vi "ProcessingLoop.vi"(8 "error in (no error)":errorcluster, 11 "navX - Base in":refnum<class "navX - Base.lvclass">) -> (0 "error out":errorcluster, 3 "navX - Base out":refnum<class "navX - Base.lvclass">)   [LabVIEW 2015, in "navX Library v3.lvlib" / "navX - Base.lvclass"]
uses:
  navX - Base.lvclass
  navX Error Status/navX Error Status.lvclass
  navX - Base.lvclass/navX - Base.ctl
  <vilib>/Platform/TimedLoop/XDataNode/timing_clust.ctl
  <vilib>/Platform/TimedLoop/XDataNode/nitl_modes.ctl
  <vilib>/Platform/TimedLoop/XDataNode/wakeup.ctl
  <vilib>/platform/TimedLoop/XDataNode/XDataNode.xnode
  <vilib>/Platform/TimedLoop/XDataNode/XDNodeRunTimeDep.lvlib
panel:
  out "Iteration Duration":i64
  out "Finished Late? [i-1]":bool
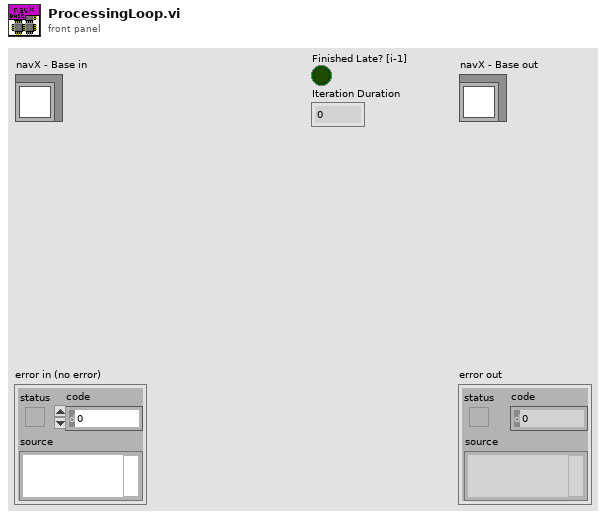
[diagram p1: front panel]
types:
  T1 = typedef "XDNodeRunTimeDep.lvlib/timing_clust.ctl" = cluster{"Expected End [f-1]":u64, "Actual End [f-1]":u64, "Finished Late? [f-1]":bool, "Expected End [i-1]":u64, "Actual End [i-1]":u64, "Finished Late? [i-1]":bool, "Expected Start [i]":u64, "Actual Start [i]":u64, "Expected Start [f]":u64, "Actual Start [f]":u64, "Source Name":string, "Structure Name":string, "Period":i64, "Deadline":i64, "Offset":i64, "Start":i64, "Priority":i32, "Timeout":i32, "Mode":T2, "Wakeup Reason":T3, "Error":errorcluster, "Source Type":string, "Secondary Source Type":string, "Global End Time":u64, "Global Start Time":u64, "Frame Duration":u64, "Iteration Duration":u64, "Assigned CPU":i32, "I/O Scan Engine Mode":u32}
  T2 = typedef "XDNodeRunTimeDep.lvlib/nitl_modes.ctl" = enum32{"No Change", "Process missed periods, maintain original phase", "Discard missed periods, maintain original phase", "Process missed periods, ignore original phase", "Discard missed periods, ignore original phase"}
  T3 = typedef "XDNodeRunTimeDep.lvlib/wakeup.ctl" = enum32{"Normal", "Aborted", "Asynchronous wakeup", "Timing source error", "Timed loop error", "Timeout"}
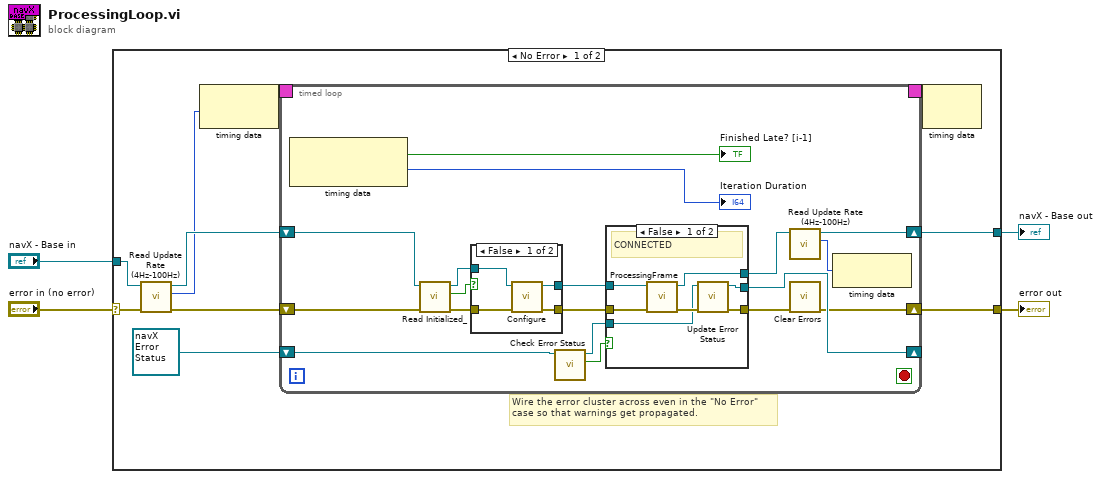
[diagram p0: block diagram]
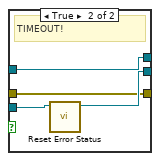
[diagram p3: hidden frame]
diagram:
  n1 = case shown="No Error" "error in (no error)" {
    selector: "error in (no error)" -> [w7 w61]
    tunnel: [w6 w61] -> w3
    tunnel: [w10 w60] -> w1
    tunnel: "navX - Base in" -> [w12 w60]
    frame No Error {
      # "Wire the error cluster across even in the \"No Error\"\ncase so that warnings get propagated."
      n2 = call "Read Update Rate (4Hz-100Hz).vi"("error in (no error)"=w7, "navX - Base in"=w12) -> ("error out"=w9:errorcluster, "Update Rate (4Hz-100Hz)"=w5:u8, "navX - Base out"=w11:refnum<class "navX - Base.lvclass">)  [unwired: 7 in]
      n3 = node-c288(w5) -> (w14:T1)
      n4 = timed-loop {
        timing: w14 -> [_]
        timing-out: [_] -> w13
        shift-right: [w32] -> w10
        shift-left: w11 -> [w21]
        shift-right: [w24] -> w6
        shift-left: w9 -> [w20]
        shift-right: [w27] -> _
        shift-left: refnum<class "navX Error Status.lvclass"> refnum ("navX Library v3.lvlib:navX Error Status.lvclass") -> [w30]
        stop <- _ stop-if-true
        n5 = node-c288() -> (→"Finished Late? [i-1]":bool, →"Iteration Duration":i64)  [unwired: 1 in]
        n6 = call "Read Initialized_.vi"("error in (no error)"=w20, "navX - Base in"=w21) -> ("error out"=w17:errorcluster, "Initialized?"=w18:bool, "navX - Base out"=w19:refnum<class "navX - Base.lvclass">)  [unwired: 7 in]
        n7 = case shown="False" w18 {
          tunnel: [w36 w37] -> w23
          tunnel: [w35 w38] -> w22
          tunnel: w19 -> [w34 w38]
          tunnel: w17 -> [w33 w37]
          frame False {
            n8 = call-dynamic "Configure.vi"("error in (no error)"=w33, "navX - Base in"=w34) -> ("error out"=w36:errorcluster, "navX - Base out"=w35:refnum<class "navX - Base.lvclass">)  [unwired: 8 in]
          }
          frame True {
          }
        }
        n9 = call "Check Error Status.vi"("navX Error Status in"=w30) -> ("Timeout!"=w29:bool, "navX Error Status out"=w28:refnum<class "navX Error Status.lvclass">)  [unwired: 8 in, 1 out]
        n10 = case shown="False" w29 {
          tunnel: w28 -> [w42 w49]
          tunnel: w22 -> [w45 w47]
          tunnel: w23 -> [w44 w46]
          tunnel: [w41 w48] -> w27
          tunnel: [w40 w46] -> w25
          tunnel: [w39 w47] -> w26
          frame False {
            # "CONNECTED"
            n11 = call-dynamic "ProcessingFrame.vi"("error in (no error)"=w44, "navX - Base in"=w45) -> ("error out"=w43:errorcluster, "navX - Base out"=w39:refnum<class "navX - Base.lvclass">)  [unwired: 8 in]
            n12 = call "Update Error Status.vi"("error in (no error)"=w43, "navX Status in"=w42) -> ("error out"=w40:errorcluster, "navX Status out"=w41:refnum<class "navX Error Status.lvclass">)  [unwired: 7 in, 1 out]
          }
          frame True {
            # "TIMEOUT!"
            n13 = call "Reset Error Status.vi"("navX Error Status in"=w49) -> ("navX Error Status out"=w48:refnum<class "navX Error Status.lvclass">)  [unwired: 9 in, 1 out]
          }
        }
        n14 = call "Read Update Rate (4Hz-100Hz).vi"("navX - Base in"=w26) -> ("Update Rate (4Hz-100Hz)"=w31:u8, "navX - Base out"=w32:refnum<class "navX - Base.lvclass">)  [unwired: 8 in, 1 out]
        n15 = call <vilib>:"Clear Errors.vi"("error in (no error)"=w25) -> ("error out"=w24:errorcluster)  [unwired: 5 in, 1 out]
        n16 = node-c288(w31) -> ()  [unwired: 1 out]
      }
      n17 = node-c288(w13) -> ()  [unwired: 1 out]
    }
    frame Error {
    }
  }
  "error out" <- w3
  "navX - Base out" <- w1
